vi "Acquire.vi"(8 "error in (no error)":errorcluster, 11 "Prototype Measurement in":refnum<class "Prototype Measurement.lvclass">) -> (0 "error out":errorcluster, 3 "Prototype Measurement out":refnum<class "Prototype Measurement.lvclass">)   [LabVIEW 2016]
uses:
  <vilib>/ActorFramework/Actor/Actor.lvclass
  user.lib/Common Components/Measurement Actor/Measurement.lvclass
  user.lib/Common Components/Measurement Actor/Messages/Measure Msg/Measure Msg.lvclass
  user.lib/Common Components/Hardware/Hardware.lvclass
  Measurement/Prototype Measurement.lvclass
  C:/Program Files (x86)/National Instruments/LabVIEW 2016/user.lib/Common Components/Measurement Actor/Measurement.lvclass
  C:/Program Files (x86)/National Instruments/LabVIEW 2016/vi.lib/ActorFramework/Actor/Actor.lvclass
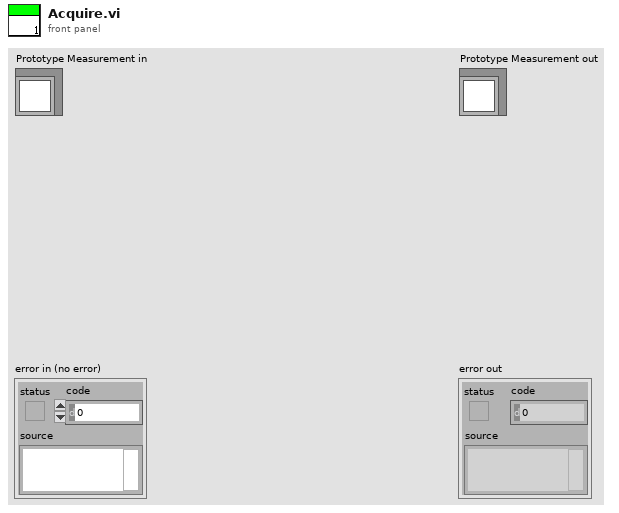
[diagram p1: front panel]
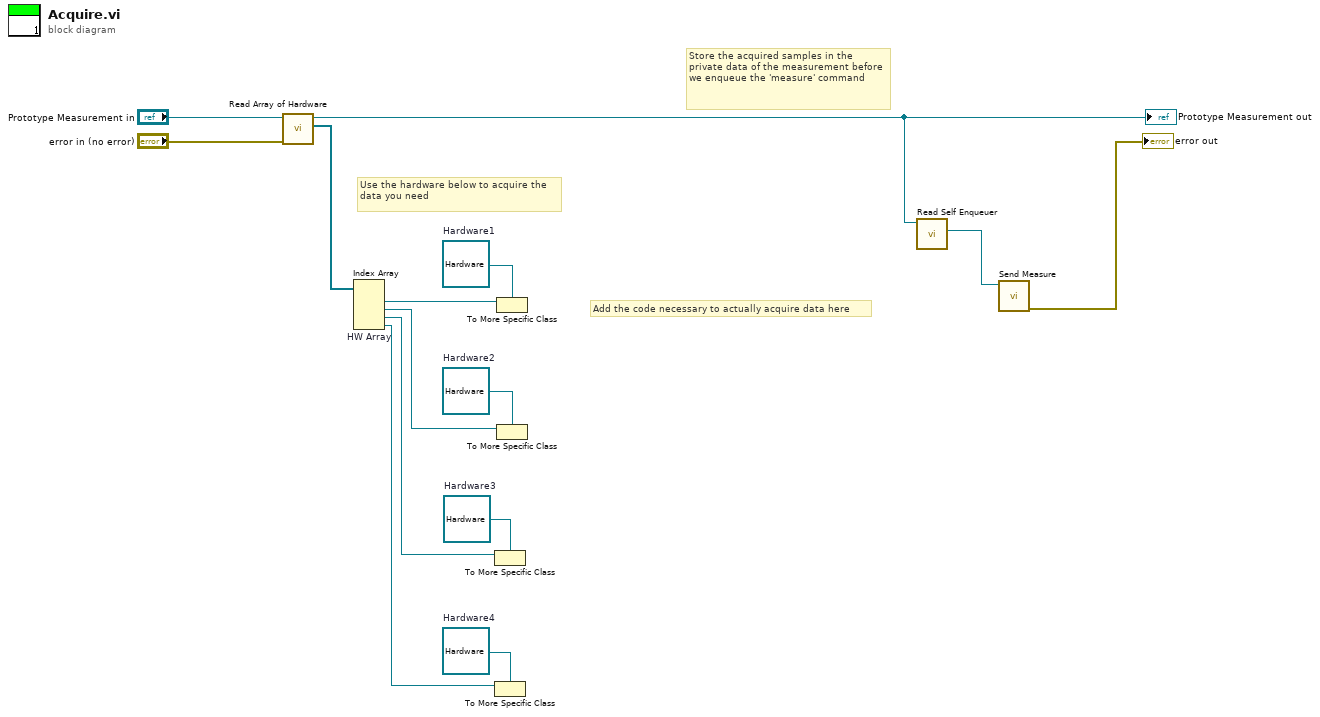
[diagram p0: block diagram]
diagram:
  w3 = refnum<class "Hardware.lvclass"> refnum  # Hardware4
  w1 = refnum<class "Hardware.lvclass"> refnum  # Hardware3
  w2 = refnum<class "Hardware.lvclass"> refnum  # Hardware2
  w4 = refnum<class "Hardware.lvclass"> refnum  # Hardware1
  # "Add the code necessary to actually acquire data here"
  # "Store the acquired samples in the private data of the measurement before we enqueue the 'measure' command"
  # "Use the hardware below to acquire the data you need"
  n1 = call "Read Array of Hardware.vi"("error in (no error)"="error in (no error)", "Measurement in"="Prototype Measurement in") -> ("Array of Hardware"=w14:refnum<class "Hardware.lvclass">[], "Measurement out"=w13:refnum<class "Prototype Measurement.lvclass">)  [unwired: 7 in, 1 out]
  "Prototype Measurement out" <- w13
  n2 = Index Array "HW Array"(array=w14) -> (element #1=w8:refnum<class "Hardware.lvclass">, element #2=w7:refnum<class "Hardware.lvclass">, element #3=w6:refnum<class "Hardware.lvclass">, element #4=w5:refnum<class "Hardware.lvclass">)  [unwired: 4 in]
  n3 = To More Specific Class ("To More Specific Class 3")(target class=w1, reference=w6) -> ()  [unwired: 1 in, 2 out]
  n4 = To More Specific Class ("To More Specific Class 4")(target class=w3, reference=w5) -> ()  [unwired: 1 in, 2 out]
  n5 = To More Specific Class ("To More Specific Class 1")(target class=w4, reference=w8) -> ()  [unwired: 1 in, 2 out]
  n6 = To More Specific Class ("To More Specific Class 2")(target class=w2, reference=w7) -> ()  [unwired: 1 in, 2 out]
  n7 = call <vilib>:"Read Self Enqueuer.vi"("Actor"=w13) -> ("Self Enqueuer"=w10:refnum<class "Message Enqueuer.lvclass">)  [unwired: 10 in]
  n8 = call "Send Measure.vi"("Message Enqueuer in"=w10) -> ("error out"=→"error out":errorcluster)  [unwired: 9 in, 1 out]
